vi "_RT_CtrlLoop_Log readFile.vi"(8 "error in":errorcluster) -> (0 "error out":errorcluster)   [LabVIEW 2018]
uses:
  <vilib>/Utility/file.llb/Read Delimited Spreadsheet (string).vi
  <vilib>/Utility/file.llb/Write Delimited Spreadsheet (string).vi
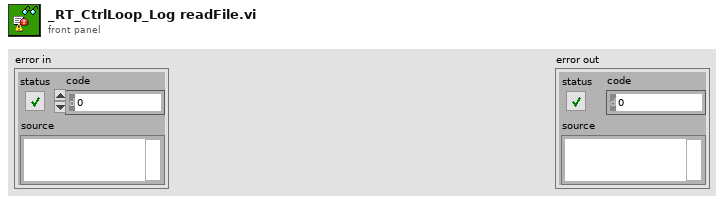
[diagram p1: front panel]
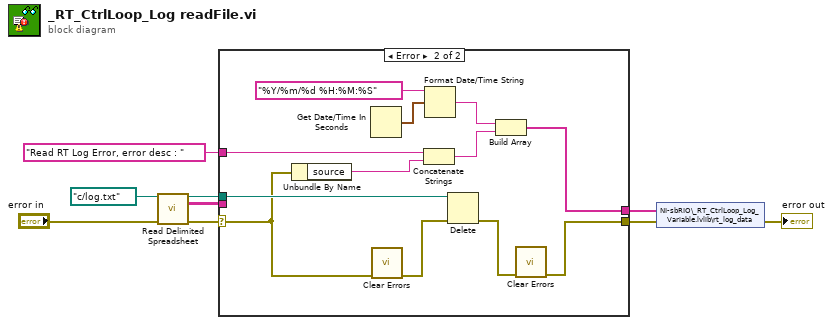
[diagram p0: block diagram]
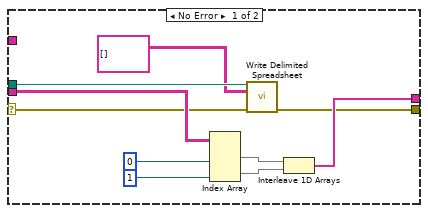
[diagram p2: hidden frame]
diagram:
  n1 = call-poly <vilib>:"Read Delimited Spreadsheet.vi"("file path (dialog if empty)"=path "c:/log.txt" ("file path (use dialog)"), "error in (no error)"="error in") -> ("new file path (Not A Path if cancelled)"=w2:path, "all rows"=w6:string[][], "error out"=w7:errorcluster)  [unwired: 8 in, 3 out]
  n2 = case shown="Error" w7 {
    selector: w7 -> [w12 w26]
    tunnel: w6 -> [w19 _]
    tunnel: [w10 w28] -> w5
    tunnel: [w14 w27] -> w4
    tunnel: w2 -> [w13 w31]
    tunnel: "Read RT Log Error, error desc : " -> [_ w25]
    frame No Error {
      n3 = Index Array(array=w19, index (col) #1=0 ("disabled index (col)"), index (col) #2=1 ("index (col)")) -> (element #1=w18:string[], element #2=w17:string[])  [unwired: 2 in]
      n4 = call-poly <vilib>:"Write Delimited Spreadsheet.vi"("file path (dialog if empty)"=w13, "2D data"=string[][] [] ("all rows"), "error in (no error)"=w12) -> ("error out"=w10:errorcluster)  [unwired: 11 in, 1 out]
      n5 = Interleave 1D Arrays(w18, w17) -> (w14:string[])
    }
    frame Error {
      n6 = Unbundle By Name(w26) -> ("source"=w24:string)
      n7 = Get Date/Time In Seconds() -> (seconds since 1Jan1904=w21:timestamp)
      n8 = call <vilib>:"Clear Errors.vi"("error in (no error)"=w26) -> ("error out"=w30:errorcluster)  [unwired: 5 in, 1 out]
      n9 = Concatenate Strings(w25, w24) -> (w23:string)
      n10 = Format Date/Time String(time format string (%c)="%Y/%m/%d %H:%M:%S", seconds (now)=w21) -> (date/time string=w20:string)  [unwired: 1 in]
      n11 = Delete(path (use dialog)=w31, error in=w30) -> (error out=w29:errorcluster)  [unwired: 3 in, 2 out]
      n12 = Build Array(w20, w23) -> (w27:string[])
      n13 = call <vilib>:"Clear Errors.vi"("error in (no error)"=w29) -> ("error out"=w28:errorcluster)  [unwired: 5 in, 1 out]
    }
  }
  n14 = shared-variable "NI-sbRIO\\_RT_CtrlLoop_Log_Variable.lvlib\\rt_log_data"(w4, error in=w5) -> (error out=→"error out":errorcluster)
